vi "NumToPercent.vi"(1 "CurVal":dbl, 2 "MinVal":dbl, 3 "MaxVal":dbl) -> (0 "IntPercent":u8)   [LabVIEW 2016]
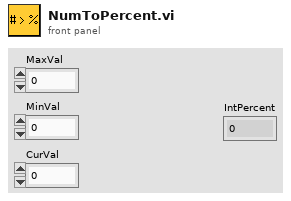
[diagram p1: front panel]
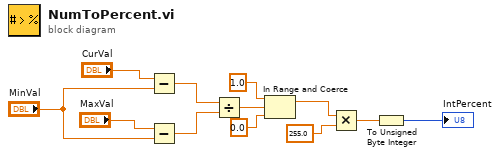
[diagram p0: block diagram]
diagram:
  n1 = Subtract(x="CurVal", y="MinVal") -> (x-y=w11:dbl)
  n2 = Subtract(x="MaxVal", y="MinVal") -> (x-y=w8:dbl)
  n3 = Divide(x=w11, y=w8) -> (x/y=w7:dbl)
  n4 = In Range and Coerce(upper limit=1.0, x=w7, lower limit=0.0) -> (coerced(x)=w4:dbl)  [unwired: 1 out]
  n5 = Multiply(x=w4, y=255.0) -> (x*y=w2:dbl)
  n6 = To Unsigned Byte Integer(number=w2) -> (unsigned 8bit integer=→"IntPercent":u8)
